vi "pouringSand.vi"(9 "sand pour":i32, 10 "Y":i32, 11 "cave":string[][](array[string])) -> (0 "escape":bool, 3 "cave":string[][](array[string]))   [LabVIEW 2025]
doc: "<b>Y</b> - start row.\n<b>sand pour</b> - column (x) from which sand is pouring."
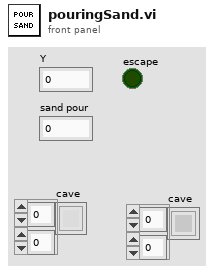
[diagram p1: front panel]
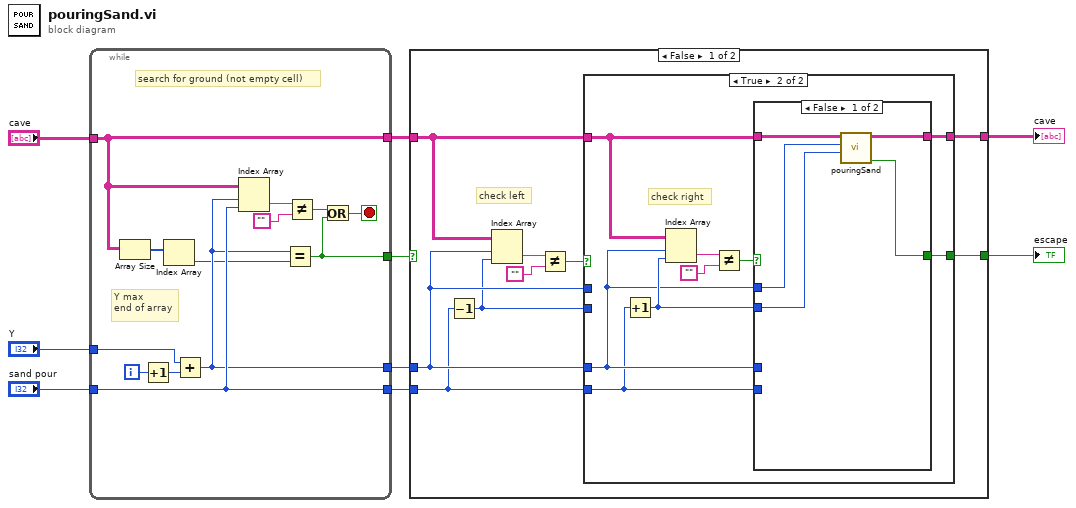
[diagram p0: block diagram]
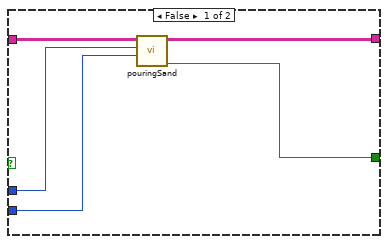
[diagram p2: hidden frame]
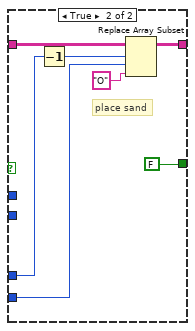
[diagram p3: hidden frame]
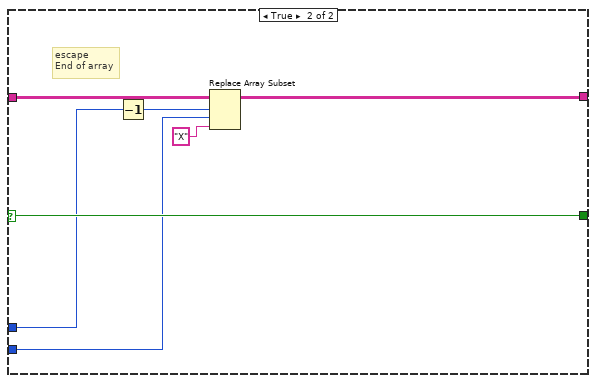
[diagram p4: hidden frame]
diagram:
  n1 = while {
    tunnel: "sand pour" -> [w16]
    tunnel: "cave" -> [w11]
    tunnel: [w14] -> w4
    tunnel: [w16] -> w3
    tunnel: [w11] -> w5
    tunnel: "Y" -> [w17]
    tunnel: [w13] -> w2
    i -> [w19]
    stop <- w15 stop-if-true
    # "Y max\nend of array"
    # "search for ground (not empty cell)"
    n2 = Array Size(array=w11) -> (size(s)=w12:i32[])
    n3 = Increment(x=w19) -> (x+1=w18:i32)
    n4 = Index Array(array=w12) -> (element=w10:i32)  [unwired: 1 in]
    n5 = Add(x=w17, y=w18) -> (x+y=w14:i32)
    n6 = Index Array(array=w11, index (row)=w14, index (col)=w16) -> (element=w22:string)
    n7 = Equal?(x=w14, y=w10) -> (x = y?=w13:bool)
    n8 = Not Equal?(x=w22, y="") -> (x != y?=w20:bool)
    n9 = Or(x=w20, y=w13) -> (x .or. y?=w15:bool)
  }
  n10 = case shown="False" w2 {
    selector: w2 -> [_ w64]
    tunnel: [w31 w60] -> w9
    tunnel: w5 -> [w28 w61]
    tunnel: w4 -> [w26 w63]
    tunnel: w3 -> [w25 w62]
    tunnel: [w23 w64] -> w1
    frame False {
      # "check left"
      n11 = Decrement(x=w25) -> (x-1=w24:i32)
      n12 = Index Array(array=w28, index (row)=w26, index (col)=w24) -> (element=w29:string)
      n13 = Not Equal?(x=w29, y="") -> (x != y?=w27:bool)
      n14 = case shown="True" w27 {
        tunnel: w28 -> [w36 w43]
        tunnel: w26 -> [_ w38]
        tunnel: w25 -> [_ w37]
        tunnel: w26 -> [w33 _]
        tunnel: w24 -> [w35 _]
        tunnel: [w34 w41] -> w31
        tunnel: [w32 w39] -> w23
        frame False {
          n15 = call "pouringSand.vi"("sand pour"=w35, "Y"=w33, "cave"=w36) -> ("escape"=w32:bool, "cave"=w34:string[][])  [unwired: 7 in]
        }
        frame True {
          # "check right"
          n16 = Increment(x=w37) -> (x+1=w40:i32)
          n17 = Index Array(array=w43, index (row)=w38, index (col)=w40) -> (element=w45:string)
          n18 = Not Equal?(x=w45, y="") -> (x != y?=w42:bool)
          n19 = case shown="False" w42 {
            tunnel: w43 -> [w48 w56]
            tunnel: w38 -> [w49 _]
            tunnel: w40 -> [w50 _]
            tunnel: w38 -> [_ w57]
            tunnel: w37 -> [_ w54]
            tunnel: [w47 w52] -> w41
            tunnel: [w46 FALSE ("Boolean")] -> w39
            frame False {
              n20 = call "pouringSand.vi"("sand pour"=w50, "Y"=w49, "cave"=w48) -> ("escape"=w46:bool, "cave"=w47:string[][])  [unwired: 7 in]
            }
            frame True {
              # "place sand"
              n21 = Decrement(x=w57) -> (x-1=w53:i32)
              n22 = Replace Array Subset(array=w56, new element="O" ("new element/subarray"), index (row)=w53, index (col)=w54) -> (w52:string[][])
            }
          }
        }
      }
    }
    frame True {
      # "escape\nEnd of array"
      n23 = Decrement(x=w63) -> (x-1=w58:i32)
      n24 = Replace Array Subset(array=w61, new element="X" ("new element/subarray"), index (row)=w58, index (col)=w62) -> (w60:string[][])
    }
  }
  "cave" <- w9
  "escape" <- w1
